vi "Write Report.vi"(8 "error in (no error)":errorcluster, 10 "Resource In":variant, 11 "Analyze Results Beam Deviation in":refnum<class "Analyze Results Beam Deviation.lvclass">) -> (0 "error out":errorcluster, 2 "Resource Out":variant, 3 "Analyze Results Beam Deviation out":refnum<class "Analyze Results Beam Deviation.lvclass">)   [LabVIEW 2020, in "Analyze Results Beam Deviation.lvclass"]
uses:
  Analyze Results Beam Deviation.lvclass
  C:/Users/AlexK/work/LabVIEW Programme/POLARIS CAM Log Abw und E/Submodules/HIJ Vision/Analyze/Results and Overlays/Results Base/Analyze Results Base.lvclass
  <vilib>/Utility/config.llb/Config Data RefNum.ctl
  Results Base/Analyze Results Base.lvclass/Analyze Results Base.ctl
  Analyze Results Beam Deviation.lvclass/Analyze Results Beam Deviation.ctl
  Results Base/Read Section.vi
  <vilib>/Utility/config.llb/Write Key (String).vi
  Results Base/Analyze Results Base.lvclass
  <vilib>/Utility/config.llb/NI_LVConfig.lvlib
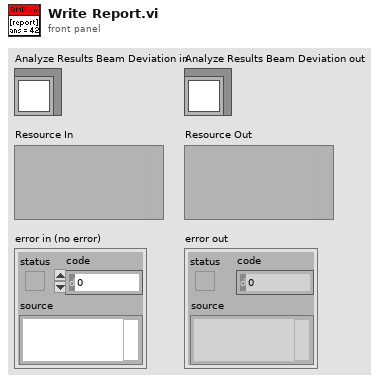
[diagram p1: front panel]
types:
  T1 = typedef "NI_LVConfig.lvlib/Config Data RefNum.ctl" = refnum<k1>
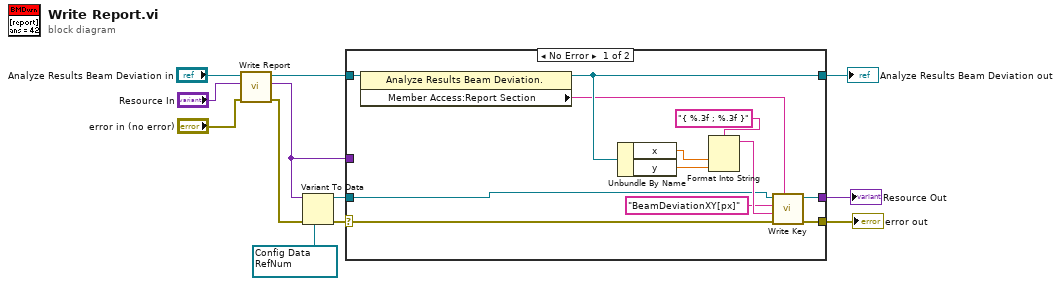
[diagram p0: block diagram]
diagram:
  w4 = T1 refnum items=["config data"] ("refnum")
  n1 = call-parent "Write Report.vi"("error in (no error)"="error in (no error)", "Resource In"="Resource In", "Analyze Results Base in"="Analyze Results Beam Deviation in") -> ("error out"=w10:errorcluster, "Resource Out"=w11:variant, "Analyze Results Base out"=w12:refnum<class "Analyze Results Beam Deviation.lvclass">)  [unwired: 6 in]
  n2 = Variant To Data(error in=w10, type=w4, Variant=w11) -> (data=w8:T1, error out=w9:errorcluster)
  n3 = case shown="No Error" w9 {
    selector: w9 -> [w20 w26]
    tunnel: w8 -> [w21 _]
    tunnel: w12 -> [w23 w25]
    tunnel: [w22 w25] -> w3
    tunnel: [w18 w27] -> w2
    tunnel: [w17 w26] -> w1
    tunnel: w11 -> [_ w27]
    frame No Error {
      n4 = property class="Analyze Results Beam Deviation."(reference=w23) -> (reference out=w22:refnum<class "Analyze Results Beam Deviation.lvclass">, "Member Access:Report Section"=w19:string)  [unwired: 1 in, 1 out]
      n5 = Unbundle By Name(w22) -> ("x"=w15:sgl, "y"=w14:sgl)
      n6 = Format Into String(format string="{ %.3f ; %.3f }", w15, w14) -> (resulting string=w24:string)  [unwired: 2 in, 1 out]
      n7 = call-poly <vilib>:"Write Key.vi"("section"=w19, "error in (no error)"=w20, "value"=w24, "key"="BeamDeviationXY[px]", "refnum"=w21) -> ("error out"=w17:errorcluster, "refnum out"=w18:T1)  [unwired: 4 in, 1 out]
    }
    frame Error {
    }
  }
  "error out" <- w1
  "Analyze Results Beam Deviation out" <- w3
  "Resource Out" <- w2
